vi "RSZVB Set Power Loss List Coefficient.vi"(6 "Transmission Coefficient (0.0)":dbl format="%^.3e", 7 "Frequency (1.0)":dbl=1.0 format="%^.3e", 8 "error in (no error)":errorcluster {"code" format="%.0x"}, 9 "Point (1)":i32=1, 10 "Operation to be Performed (Insert)":i32(ring) items=["Insert", "Append"], 11 "VISA session":refnum<visa-resource-name>) -> (0 "error out":errorcluster {"code" format="%.0x"}, 3 "dup VISA session":refnum<visa-resource-name>)   [LabVIEW 2011]
doc: "This VI Adds a new frequency and transmission coefficient to the power loss list.\n\nRemote-control command(s):\nSOURce<Ch>:POWer<Pt>:CORRection:TCOefficient:DEFine <frequency>, <transmission>\nSOURce<Ch>:POWer<Pt>:CORRection:TCOefficient:INSert<List_No>\n<frequency>, <transmission>"
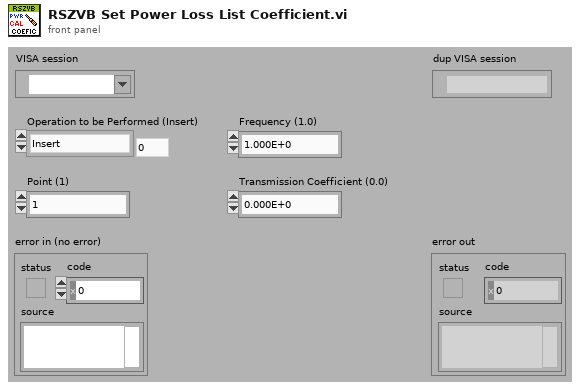
[diagram p1: front panel]
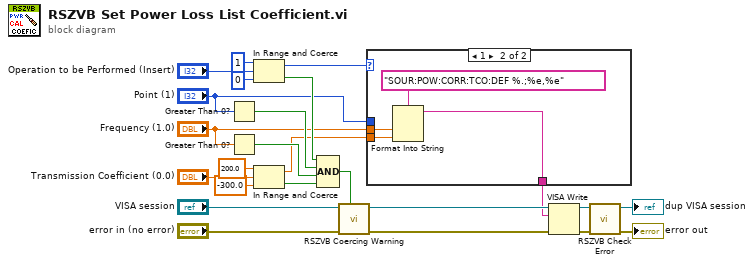
[diagram p0: block diagram]
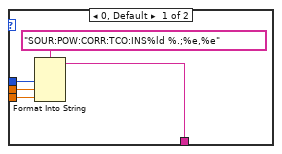
[diagram p2: hidden frame]
diagram:
  n1 = Greater Than 0?(x="Point (1)") -> (x > 0?=w11:bool)
  n2 = Greater Than 0?(x="Frequency (1.0)") -> (x > 0?=w10:bool)
  n3 = In Range and Coerce(upper limit=1, x="Operation to be Performed (Insert)", lower limit=0) -> (coerced(x)=w7:i32, In Range?=w12:bool)
  n4 = In Range and Coerce(upper limit=200.0, x="Transmission Coefficient (0.0)", lower limit=-300.0) -> (coerced(x)=w4:dbl, In Range?=w9:bool)
  n5 = Compound Arithmetic op=AND(w12, w11, w10, w9) -> (w8:bool)
  n6 = call "RSZVB Coercing Warning.vi"("In Range?"=w8, "error in (no error)"="error in (no error)", "VISA session"="VISA session") -> ("error out"=w23:errorcluster, "dup VISA session"=w24:refnum<visa-resource-name>)  [unwired: 7 in]
  n7 = case shown="1" w7 {
    tunnel: "Point (1)" -> [w28 _]
    tunnel: "Frequency (1.0)" -> [w27 w32]
    tunnel: w4 -> [w26 w31]
    tunnel: [w25 w30] -> w1
    frame 0, Default {
      n8 = Format Into String(format string="SOUR:POW:CORR:TCO:INS%ld %.;%e,%e", w28, w27, w26) -> (resulting string=w25:string)  [unwired: 2 in, 1 out]
    }
    frame 1 {
      n9 = Format Into String(format string="SOUR:POW:CORR:TCO:DEF %.;%e,%e", w32, w31) -> (resulting string=w30:string)  [unwired: 2 in, 1 out]
    }
  }
  n10 = VISA Write(VISA resource name=w24, write buffer=w1, error in (no error)=w23) -> (VISA resource name out=w21:refnum<visa-resource-name>, error out=w22:errorcluster)  [unwired: 1 out]
  n11 = call "RSZVB Check Error.vi"("error in (no error)"=w22, "VISA session"=w21) -> ("error out"=→"error out":errorcluster, "dup VISA session"=→"dup VISA session":refnum<visa-resource-name>)  [unwired: 8 in]
